vi "testtesattest.vi"() -> ()   [LabVIEW 2019]
panel:
  out "data 3":dbl
  out "data 2":bool
  out "data":dbl
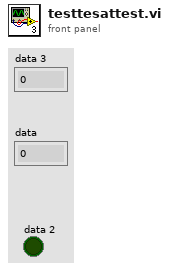
[diagram p1: front panel]
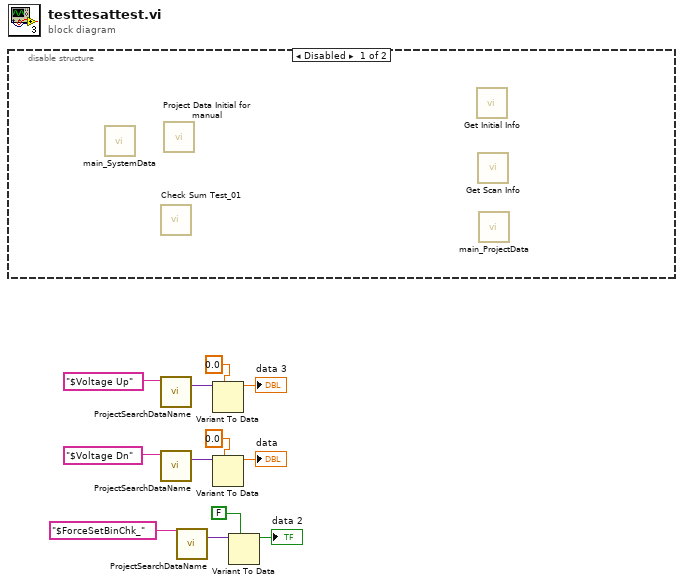
[diagram p0: block diagram]
diagram:
  n1 = disable-structure shown="Disabled" {
    frame Disabled {
      n2 = call "main_SystemData.vi"() -> ()  [unwired: 9 in, 3 out]
      n3 = call "Check Sum Test_01.vi"() -> ()  [unwired: 9 in, 3 out]
      n4 = call "Project Data Initial for manual.vi"() -> ()  [unwired: 8 in, 4 out]
      n5 = call "Get Initial Info.vi"() -> ()  [unwired: 10 in, 2 out]
      n6 = call "Get Scan Info.vi"() -> ()  [unwired: 10 in, 2 out]
      n7 = call "main_ProjectData.vi"() -> ()  [unwired: 9 in, 3 out]
    }
    frame Enabled {
    }
  }
  n8 = call "ProjectSearchDataName.vi"("element"="$Voltage Up") -> ("variant"=w2:variant)  [unwired: 8 in, 2 out]
  n9 = call "ProjectSearchDataName.vi"("element"="$Voltage Dn") -> ("variant"=w11:variant)  [unwired: 8 in, 2 out]
  n10 = call "ProjectSearchDataName.vi"("element"="$ForceSetBinChk_") -> ("variant"=w8:variant)  [unwired: 8 in, 2 out]
  n11 = Variant To Data(type=0.0, Variant=w2) -> (data=→"data 3":dbl)  [unwired: 1 in, 1 out]
  n12 = Variant To Data(type=0.0, Variant=w11) -> (data=→"data":dbl)  [unwired: 1 in, 1 out]
  n13 = Variant To Data(type=FALSE, Variant=w8) -> (data=→"data 2":bool)  [unwired: 1 in, 1 out]
